vi "DDS Channel to Master Reset Pin.vi"(1 "channel number (1)":u8=1 min=1 max=4 step=1) -> (0 "DIO pin":T1)   [LabVIEW 2013]
doc: "Given a channel number, returns the enum representing the channel's master reset DIO pin."
uses:
  DDS DIO pins.ctl
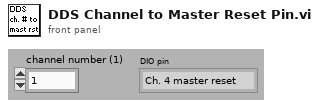
[diagram p1: front panel]
types:
  T1 = typedef "DDS DIO pins.ctl" = enum8{"Ch. 4 master reset", "Ch. 3 master reset", "Ch. 2 master reset", "Ch. 1 master reset", "Ch. 1 IO update", "Ch. 2 IO update", "Ch. 3 IO update", "Ch. 4 IO update"}
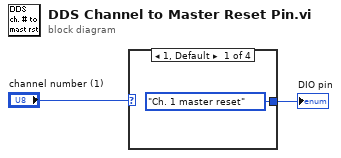
[diagram p0: block diagram]
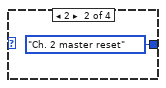
[diagram p2: hidden frame]
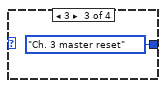
[diagram p3: hidden frame]
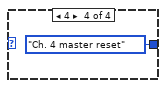
[diagram p4: hidden frame]
diagram:
  n1 = case shown="1, Default" "channel number (1)" {
    tunnel: [DDS_DIO_pins."Ch. 1 master reset" ("DDS DIO pins") DDS_DIO_pins."Ch. 2 master reset" ("DDS DIO pins") DDS_DIO_pins."Ch. 3 master reset" ("DDS DIO pins") DDS_DIO_pins."Ch. 4 master reset" ("DDS DIO pins")] -> w1
    frame 1, Default {
    }
    frame 2 {
    }
    frame 3 {
    }
    frame 4 {
    }
  }
  "DIO pin" <- w1
